vi "Set.vi"(0 "VISA resource name":refnum<visa-resource-name>, 1 "Local Lockout (0:1)":u32(ring) items=["Off", "On"], 2 "ATTN (0:1)":u32(ring) items=["Off", "On"], 3 "Run/Stop (1:0)":u32(ring)=1 items=["Stop", "Run"], 5 "Wavelength (nnnn)":dbl[unit]=8.210000000000001e-07, 6 "AVG (1:3)":u32(ring)=2 items=["Slow"=1, "Medium"=2, "Fast"=3], 9 "Range (0-Auto,1:8)":u32(ring) items=["Auto", "Lowest", "2", "3", "4", "5", "6", "7", "Highest"], 10 "Units (1:4)":u32(ring)=1 items=["W"=1, "dB"=2, "dBm"=3, "REL"=4], 11 "error in (no error)":errorcluster, 12 "Backlight (0:2)":u32(ring)=1 items=["Off", "Low", "High"], 13 "Beeper (0:1)":u32(ring) items=["Off", "On"], 14 "Zero (0:1)":u32(ring) items=["Off", "On"]) -> (4 "VISA resource name out":refnum<visa-resource-name>, 15 "error out":errorcluster)   [LabVIEW 2017]
doc: "Sets 1830-C options in succession."
uses:
  <vilib>/Utility/error.llb/DialogType.ctl
  Newport 1830-C/Newport 1830-C.lvlib
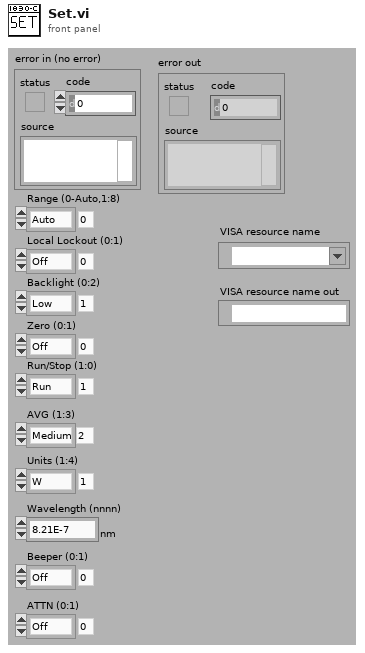
[diagram p1: front panel]
types:
  T1 = typedef "DialogType.ctl" = u16
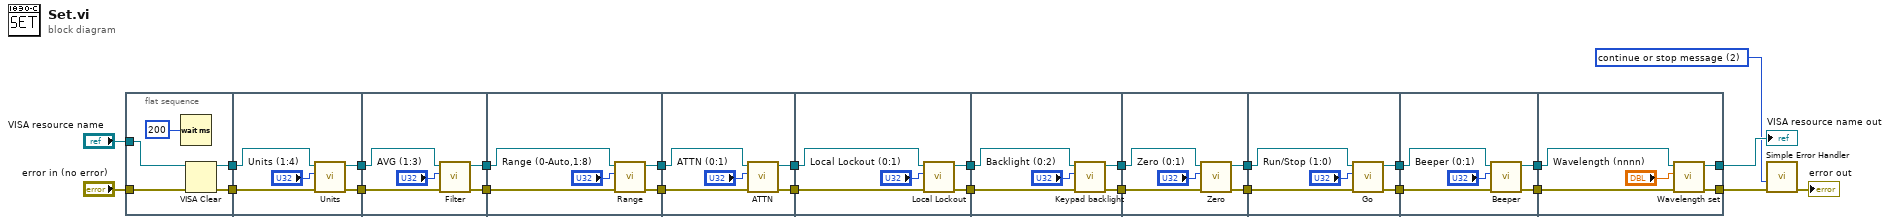
[diagram p0: block diagram]
diagram:
  w1 = T1 2 items=["no dialog", "OK message", "continue or stop message", "OK message + warnings", "continue/stop + warnings"] ("type of dialog (OK msg:1)")
  n1 = flat-sequence {
    tunnel: "error in (no error)" -> [w28]
    tunnel: "VISA resource name" -> [w29]
    tunnel: [w31] -> w5
    tunnel: [w30] -> w4
    tunnel: [w34] -> w25
    tunnel: [w32] -> w14
    tunnel: w5 -> [w35]
    tunnel: w4 -> [w33]
    tunnel: w25 -> [w40]
    tunnel: [w39] -> w23
    tunnel: w14 -> [w38]
    tunnel: [w37] -> w13
    tunnel: w23 -> [w45]
    tunnel: [w44] -> w22
    tunnel: w13 -> [w43]
    tunnel: [w42] -> w12
    tunnel: w22 -> [w50]
    tunnel: [w49] -> w21
    tunnel: w12 -> [w48]
    tunnel: [w47] -> w11
    tunnel: w21 -> [w55]
    tunnel: [w54] -> w20
    tunnel: w11 -> [w53]
    tunnel: [w52] -> w10
    tunnel: w20 -> [w60]
    tunnel: [w59] -> w19
    tunnel: w10 -> [w58]
    tunnel: [w57] -> w9
    tunnel: w19 -> [w65]
    tunnel: [w64] -> w18
    tunnel: w9 -> [w63]
    tunnel: [w62] -> w8
    tunnel: w18 -> [w70]
    tunnel: [w69] -> w17
    tunnel: w8 -> [w68]
    tunnel: [w67] -> w7
    tunnel: w17 -> [w75]
    tunnel: [w74] -> w16
    tunnel: w7 -> [w73]
    tunnel: [w72] -> w6
    tunnel: w16 -> [w80]
    tunnel: [w79] -> w15
    tunnel: [w78] -> w2
    tunnel: w6 -> [w77]
    frame #0 {
      n2 = Wait (ms)(milliseconds to wait=u32 200) -> ()  [unwired: 1 out]
      n3 = VISA Clear(VISA resource name=w29, error in (no error)=w28) -> (VISA resource name out=w31:refnum<visa-resource-name>, error out=w30:errorcluster)
    }
    frame #1 {
      n4 = call "Units.vi"("error in (no error)"=w33, "Units"="Units (1:4)", "VISA resource name"=w35) -> ("error out"=w32:errorcluster, "VISA resource name out"=w34:refnum<visa-resource-name>)  [unwired: 7 in]
    }
    frame #2 {
      n5 = call "Filter.vi"("error in (no error)"=w38, "Filter"="AVG (1:3)", "VISA resource name"=w40) -> ("error out"=w37:errorcluster, "VISA resource name out"=w39:refnum<visa-resource-name>)  [unwired: 7 in]
    }
    frame #3 {
      n6 = call "Range.vi"("error in (no error)"=w43, "Range"="Range (0-Auto,1:8)", "VISA resource name"=w45) -> ("error out"=w42:errorcluster, "VISA resource name out"=w44:refnum<visa-resource-name>)  [unwired: 7 in]
    }
    frame #4 {
      n7 = call "ATTN.vi"("error in (no error)"=w48, "Attn"="ATTN (0:1)", "VISA resource name"=w50) -> ("error out"=w47:errorcluster, "VISA resource name out"=w49:refnum<visa-resource-name>)  [unwired: 7 in]
    }
    frame #5 {
      n8 = call "Local Lockout.vi"("error in (no error)"=w53, "Local Lockout"="Local Lockout (0:1)", "VISA resource name"=w55) -> ("error out"=w52:errorcluster, "VISA resource name out"=w54:refnum<visa-resource-name>)  [unwired: 7 in]
    }
    frame #6 {
      n9 = call "Keypad backlight.vi"("error in (no error)"=w58, "BKLT"="Backlight (0:2)", "VISA resource name"=w60) -> ("error out"=w57:errorcluster, "VISA resource name out"=w59:refnum<visa-resource-name>)  [unwired: 7 in]
    }
    frame #7 {
      n10 = call "Zero.vi"("error in (no error)"=w63, "Zero"="Zero (0:1)", "VISA resource name"=w65) -> ("error out"=w62:errorcluster, "VISA resource name out"=w64:refnum<visa-resource-name>)  [unwired: 7 in]
    }
    frame #8 {
      n11 = call "Go.vi"("error in (no error)"=w68, "Run/Stop"="Run/Stop (1:0)", "VISA resource name"=w70) -> ("error out"=w67:errorcluster, "VISA resource name out"=w69:refnum<visa-resource-name>)  [unwired: 7 in]
    }
    frame #9 {
      n12 = call "Beeper.vi"("error in (no error)"=w73, "Beeper"="Beeper (0:1)", "VISA resource name"=w75) -> ("error out"=w72:errorcluster, "VISA resource name out"=w74:refnum<visa-resource-name>)  [unwired: 7 in]
    }
    frame #10 {
      n13 = call "Wavelength set.vi"("error in (no error)"=w77, "Wavelength (nnnn)"="Wavelength (nnnn)", "VISA resource name"=w80) -> ("error out"=w78:errorcluster, "VISA resource name out"=w79:refnum<visa-resource-name>)  [unwired: 7 in]
    }
  }
  n14 = call <vilib>:"Simple Error Handler.vi"("type of dialog (OK msg:1)"=w1, "error in (no error)"=w2) -> ("error out"=→"error out":errorcluster)  [unwired: 3 in, 4 out]
  "VISA resource name out" <- w15
